vi "drawField.vi"(0 "Vision in":refnum<class "Vision.lvclass">, 1 "AutoScale":bool=TRUE, 2 "Game reference":refnum<data-value>, 5 "Field State Input":T1 {"Detection Frame Out"."robots_blue"."height" format="%+4.3f"; "Detection Frame Out"."robots_blue"."pixel_y" format="%+4.3f"; "Detection Frame Out"."robots_blue"."pixel_x" format="%+4.3f"; "Detection Frame Out"."robots_blue"."orientation" format="%+4.3f"; "Detection Frame Out"."robots_blue"."y" format="%+4.3f"; "Detection Frame Out"."robots_blue"."confidence" format="%4.3f"; "Detection Frame Out"."robots_blue"."x" format="%+4.3f"; "Detection Frame Out"."robots_yellow"."height" format="%+4.3f"; "Detection Frame Out"."robots_yellow"."pixel_y" format="%+4.3f"; "Detection Frame Out"."robots_yellow"."pixel_x" format="%+4.3f"; "Detection Frame Out"."robots_yellow"."orientation" format="%+4.3f"; "Detection Frame Out"."robots_yellow"."y" format="%+4.3f"; "Detection Frame Out"."robots_yellow"."confidence" format="%4.3f"; "Detection Frame Out"."robots_yellow"."x" format="%+4.3f"}, 11 "error in (no error)":errorcluster, 12 "Scale mm/pixel":dbl=0.094076928 format="%#_13g", 13 "Draw Targets?":T6, 14 "Zoom":dbl) -> (3 "AutoScale Out":bool=TRUE, 4 "Vision out":refnum<class "Vision.lvclass">, 6 "2D Picture":picture, 10 "Scale Out":dbl, 15 "error out":errorcluster)   [LabVIEW 2021, in "Vision.lvclass"]
uses:
  Vision.lvclass
  DrawTargets.ctl
  Controls/SSL Field State.ctl
  Controls/SSL Detection Frame.ctl
  Controls/SSL Detection Robot.ctl
  <vilib>/Analysis/Matrix/Datatypes/RealMatrix.ctl
  Controls/SSL Detection Ball.ctl
  Game_class/Game.lvclass
  <vilib>/Utility/miscctls.llb/LVBoundsTypeDef.ctl
  Robot_class/Robot.lvclass
  Game_class/Game.lvclass/Game.ctl
  Team_class/Team.lvclass/Team.ctl
  Parameters_class/Parameters.lvclass/Parameters.ctl
  Game_class/Read Referee.vi
  Game_class/Read OffensiveTeam.vi
  Game_class/Read DefensiveTeam.vi
  Game_class/Read KeeperTeam.vi
  Game_class/Read Parameters.lvclass.vi
  Game_class/Read FieldRef.vi
  Game_class/Read AllyRef.vi
  Game_class/Read EnemyRef.vi
  Game_class/Read BallRef.vi
  Team_class/Read RobotRef.vi
  Parameters_class/Read Area.vi
  Parameters_class/Read Project.vi
  Team_class/Read KeeperPlay.vi
  Ally_class/Ally.lvclass
  D:/RoboIme/horie/SSL_AI/Team_class/Team.lvclass
  Enemy_class/Enemy.lvclass
  Referee_class/Referee.lvclass
  Parameters_class/Parameters.lvclass
  Field_class/Field.lvclass
  Ball_class/Ball.lvclass
  <vilib>/Analysis/Matrix/NI_Matrix.lvlib
panel:
  in  "Defense stretch":i32=500
  in  "Draw Number":bool=TRUE
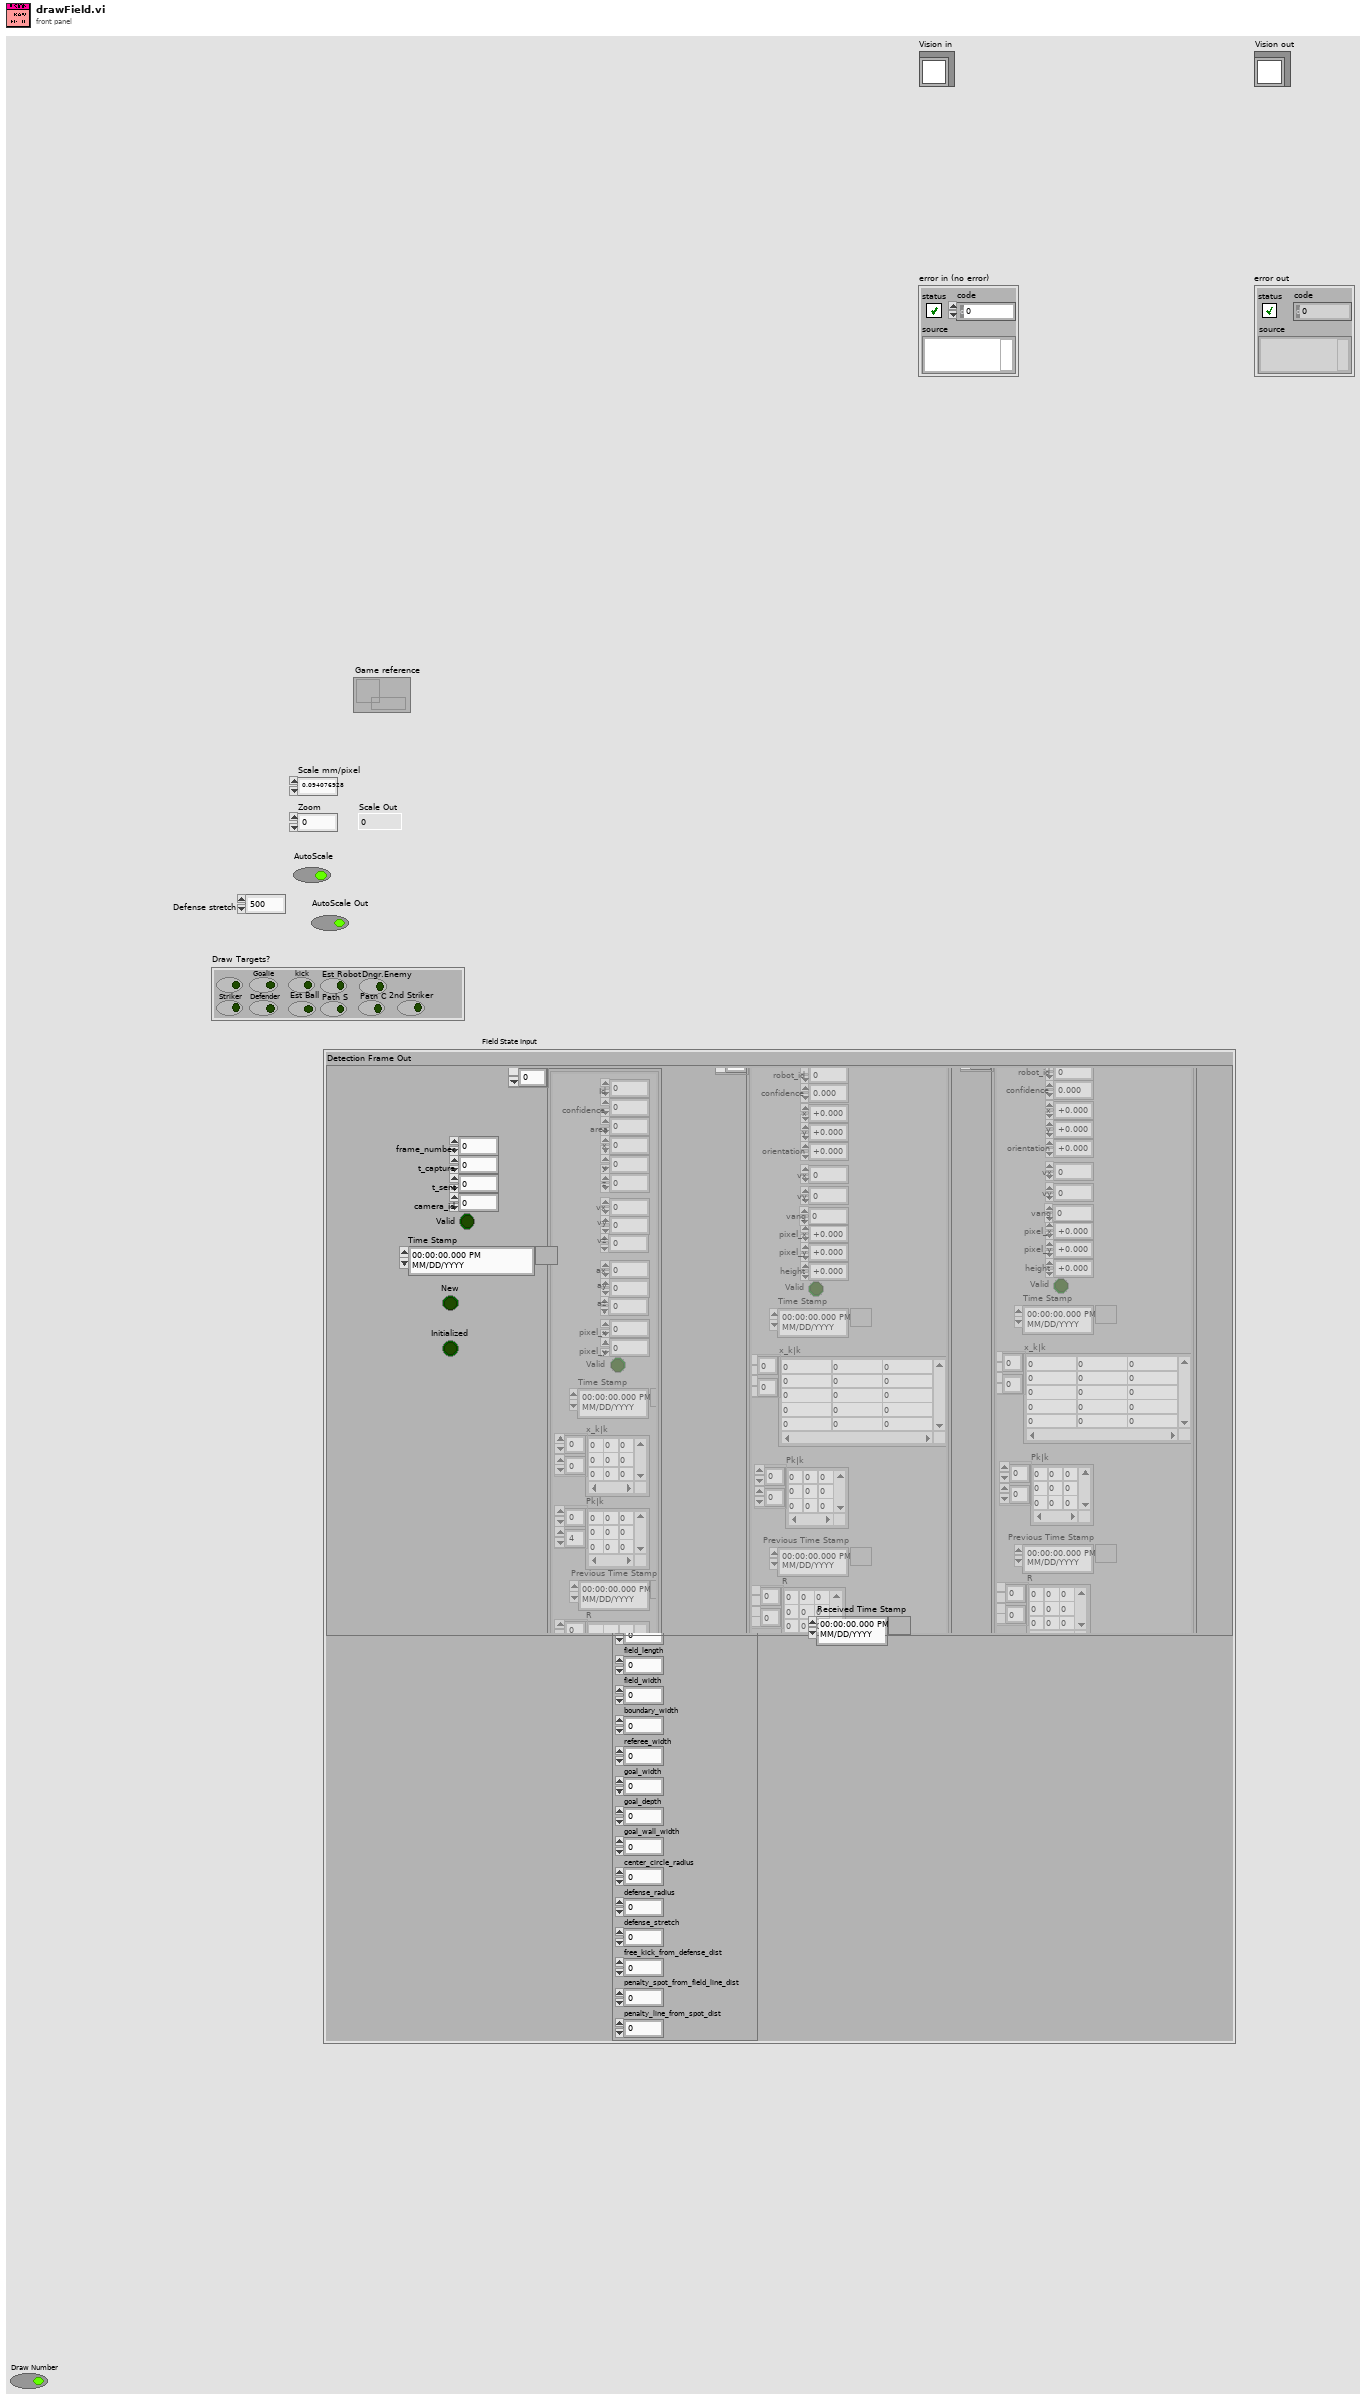
[diagram p1: front panel]
types:
  T1 = typedef "SSL Field State.ctl" = cluster{"Detection Frame Out":T2, "Field Size Out":cluster{"line_width":u32, "field_length":u32, "field_width":u32, "boundary_width":u32, "referee_width":u32, "goal_width":u32, "goal_depth":u32, "goal_wall_width":u32, "center_circle_radius":u32, "defense_radius":u32, "defense_stretch":u32, "free_kick_from_defense_dist":u32, "penalty_spot_from_field_line_dist":u32, "penalty_line_from_spot_dist":u32}, "Received Time Stamp":timestamp}
  T2 = typedef "SSL Detection Frame.ctl" = cluster{"frame_number":u32, "t_capture":dbl, "t_sent":dbl, "camera_id":u32, "robots_yellow":T3[], "robots_blue":T3[], "balls":T5[], "Valid":bool, "Time Stamp":timestamp, "New":bool, "Initialized":bool}
  T3 = typedef "SSL Detection Robot.ctl" = cluster{"x":sgl, "robot_id":u32, "confidence":sgl, "y":sgl, "orientation":sgl, "pixel_x":sgl, "pixel_y":sgl, "height":sgl, "Valid":bool, "Time Stamp":timestamp, "x_k|k":T4, "Pk|k":T4, "Previous Time Stamp":timestamp, "R":T4, "vx":dbl, "vy":dbl, "vang":dbl}
  T4 = typedef "NI_Matrix.lvlib/RealMatrix.ctl" = dbl[][]
  T5 = typedef "SSL Detection Ball.ctl" = cluster{"x":sgl, "area":u32, "confidence":sgl, "y":sgl, "z":sgl, "pixel_x":sgl, "pixel_y":sgl, "Valid":bool, "Time Stamp":timestamp, "x_k|k":T4, "Pk|k":T4, "Id":u32, "Previous Time Stamp":timestamp, "R":T4, " vx":sgl, "vy":dbl, "vz":dbl, " ax":sgl, "ay":dbl, "az":dbl}
  T6 = typedef "DrawTargets.ctl" = cluster{"Attacker":bool, "Striker":bool, "Goalie":bool, "Defender":bool, "kick":bool, "Est Ball":bool, "Est Robot":bool, "Path S":bool, "Path C":bool, "Dngr.Enemy":bool, "2nd Striker":bool}
  T7 = typedef "LVBoundsTypeDef.ctl" = cluster{"Width":u32, "Height":u32}
  T8 = typedef "Project.ctl" = enum16{"SSL", "VSS"}
  T9 = typedef "KeeperPlay.ctl" = enum16{"SimpleBallPlacementAlly", "BallPlacementAlly", "BallPlacementEnemy", "ZigZag", "Goto", "NormalGame", "KeeperPlay", "Halt", "Timeout", "PenaltyEnemy", "TestPlay"}
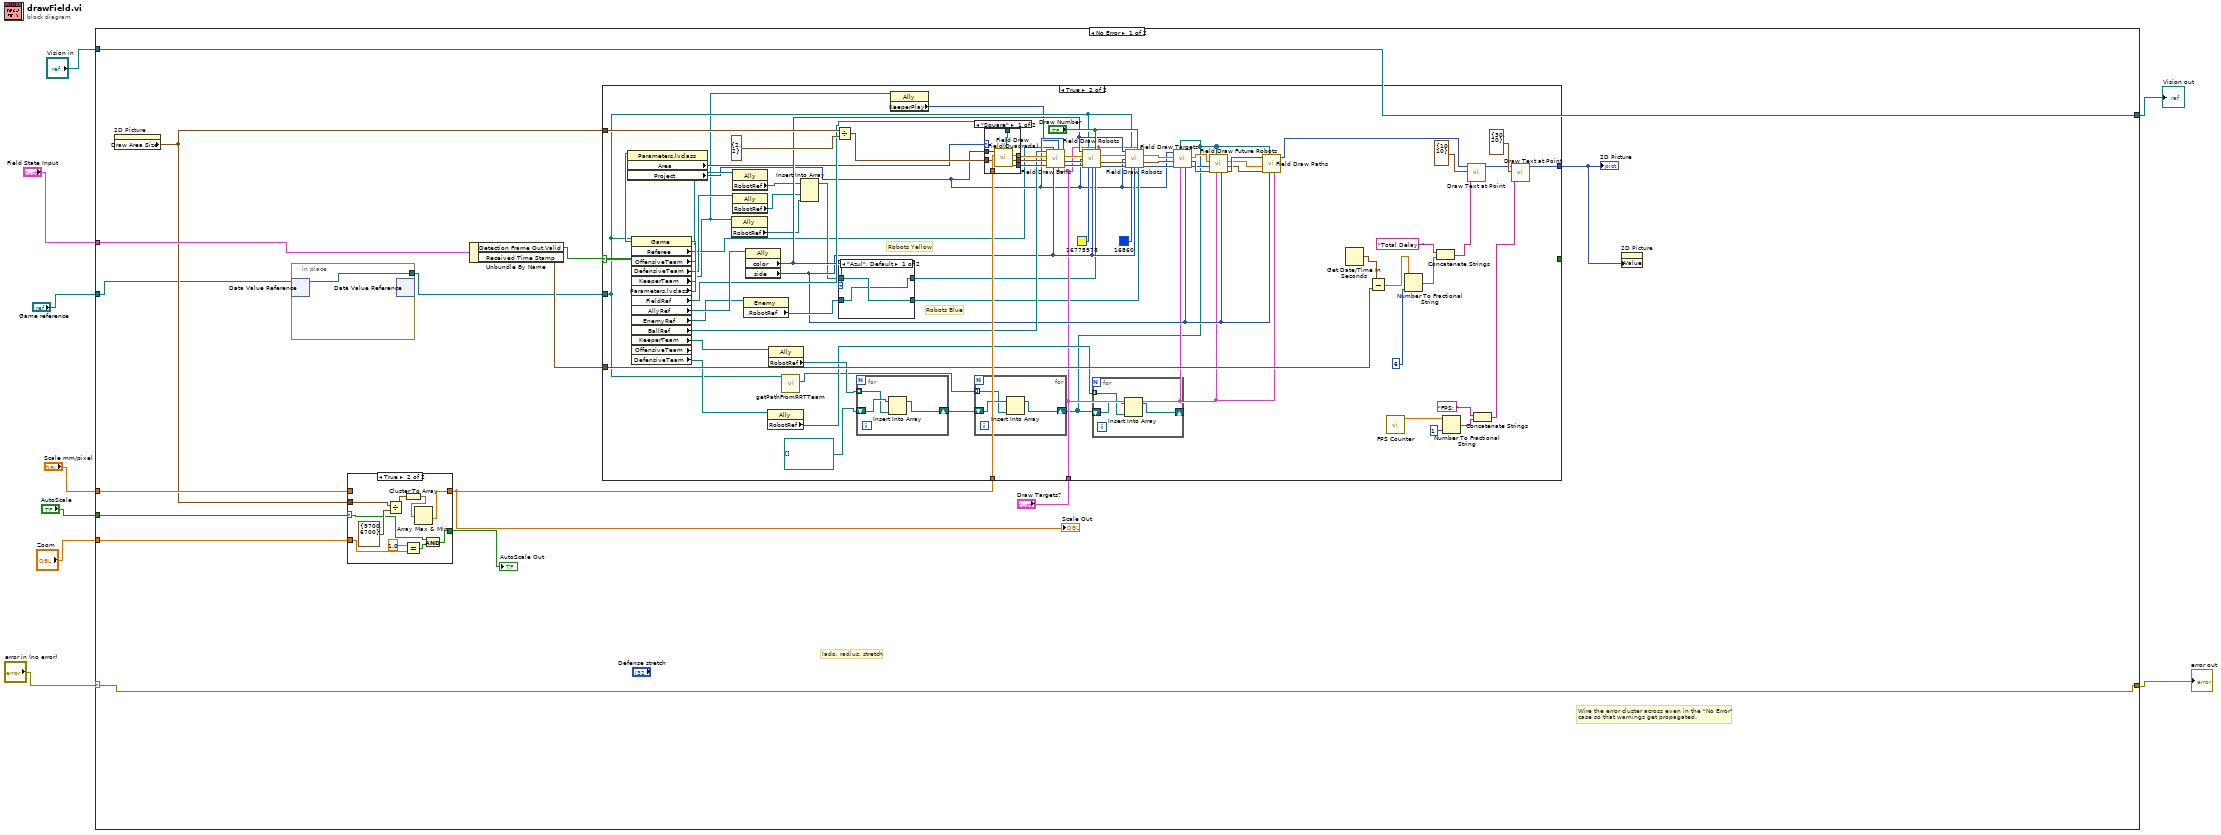
[diagram p0: block diagram]
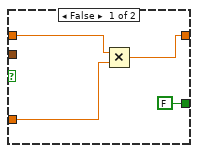
[diagram p2: hidden frame]
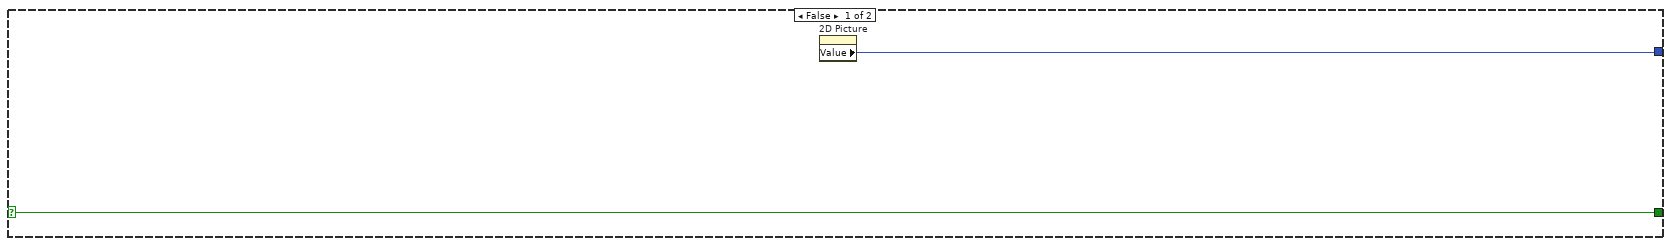
[diagram p3: hidden frame]
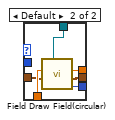
[diagram p5: hidden frame]
diagram:
  n1 = case shown="No Error" "error in (no error)" {
    selector: "error in (no error)" -> [w23 w142]
    tunnel: [w23 w142] -> w8
    tunnel: [w24 w141] -> w6
    tunnel: "Vision in" -> [w24 w141]
    tunnel: "Scale mm/pixel" -> [w20 _]
    tunnel: "AutoScale" -> [w19 _]
    tunnel: "Zoom" -> [w18 _]
    tunnel: "Field State Input" -> [w16 _]
    tunnel: "Game reference" -> [w13 _]
    frame No Error {
      # "lado, radius, stretch"
      # "Wire the error cluster across even in the \"No Error\"\ncase so that warnings get propagated."
      n2 = property on="2D Picture" class="Pict"() -> ("Draw Area Size"=w15:T7)  [unwired: 2 in, 2 out]
      n3 = in-place {
        in-place-border: [w25] -> w12
        n4 = in-place-dvr #1(w13) -> (w25:refnum<class "Game.lvclass">)  [unwired: 1 out]
        n5 = in-place-dvr #1() -> ()  [unwired: 1 in, 2 out]
      }
      n6 = case shown="True" w19 {
        selector: w19 -> [_ w31]
        tunnel: w20 -> [w29 _]
        tunnel: [w28 w35] -> w14
        tunnel: w15 -> [_ w39]
        tunnel: w18 -> [w27 w34]
        tunnel: [FALSE w32] -> w17
        frame False {
          n7 = Multiply(x=w29, y=w27) -> (x*y=w28:dbl)
        }
        frame True {
          n8 = Divide(x=w39, y=T7 {"Width"=9700, "Height"=6700}) -> (x/y=w37:cluster{"Width":dbl, "Height":dbl})
          n9 = Cluster To Array(cluster=w37) -> (array=w36:dbl[])
          n10 = Equal?(x=1.0, y=w34) -> (x = y?=w30:bool)
          n11 = Array Max & Min(array=w36) -> (min value=w35:dbl)  [unwired: 3 out]
          n12 = And(x=w31, y=w30) -> (x .and. y?=w32:bool)
        }
      }
      "Scale Out" <- w14
      "AutoScale Out" <- w17
      n13 = Unbundle By Name(w16) -> ("Detection Frame Out.Valid"=w11:bool, "Received Time Stamp"=w22:timestamp)
      n14 = case shown="True" w11 {
        selector: w11 -> [w41 _]
        tunnel: w15 -> [_ w113]
        tunnel: [w40 w94] -> w10
        tunnel: w14 -> [_ w106]
        tunnel: [w41 _] -> _
        tunnel: w22 -> [_ w101]
        tunnel: "Draw Targets?" -> [_ w59]
        tunnel: w12 -> [_ w46]
        frame False {
          n15 = property on="2D Picture" class="Pict"() -> ("Value"=w40:picture)  [unwired: 2 in, 2 out]
        }
        frame True {
          # "Robots Blue"
          # "Robots Yellow"
          n16 = property class="Game" props=["Referee", "OffensiveTeam", "DefensiveTeam", "KeeperTeam", "Parameters.lvclass", "FieldRef", "AllyRef", "EnemyRef", "BallRef", "KeeperTeam", "OffensiveTeam", "DefensiveTeam"](reference=w46) -> ("Referee"=w44:refnum<class "Referee.lvclass">, "OffensiveTeam"=w56:refnum<class "Ally.lvclass">, "DefensiveTeam"=w55:refnum<class "Ally.lvclass">, "KeeperTeam"=w43:refnum<class "Ally.lvclass">, "Parameters.lvclass"=w61:refnum<class "Parameters.lvclass">, "FieldRef"=w70:refnum<class "Field.lvclass">, "AllyRef"=w76:refnum<class "Ally.lvclass">, "EnemyRef"=w75:refnum<class "Enemy.lvclass">, "BallRef"=w73:refnum<class "Ball.lvclass">, "KeeperTeam"=w68:refnum<class "Ally.lvclass">, "DefensiveTeam"=w67:refnum<class "Ally.lvclass">)  [unwired: 1 in, 3 out]
          n17 = property class="Parameters.lvclass"(reference=w61) -> ("Area"=w60:enum16{"Circular", "Square"}, "Project"=w48:T8)  [unwired: 1 in, 2 out]
          n18 = property class="Ally"(reference=w43) -> ("RobotRef"=w52:refnum<class "Robot.lvclass">[])  [unwired: 1 in, 2 out]
          n19 = property class="Ally"(reference=w56) -> ("RobotRef"=w54:refnum<class "Robot.lvclass">[])  [unwired: 1 in, 2 out]
          n20 = property class="Ally"(reference=w55) -> ("RobotRef"=w53:refnum<class "Robot.lvclass">[])  [unwired: 1 in, 2 out]
          n21 = property class="Enemy"(reference=w75) -> ("RobotRef"=w74:refnum<class "Robot.lvclass">[])  [unwired: 1 in, 2 out]
          n22 = property class="Ally"(reference=w76) -> ("color"=w69:enum16{"Azul", "Amarelo"}, "side"=w62:enum16{"Esquerdo", "Direito"})  [unwired: 1 in, 2 out]
          n23 = property class="Ally"(reference=w67) -> ("RobotRef"=w63:refnum<class "Robot.lvclass">[])  [unwired: 1 in, 2 out]
          n24 = property class="Ally"(reference=w68) -> ("RobotRef"=w64:refnum<class "Robot.lvclass">[])  [unwired: 1 in, 2 out]
          n25 = call "getPathFromRRTTeam.vi"("Game in"=w46) -> ("RoboRef"=w47:refnum<class "Robot.lvclass">[])  [unwired: 8 in, 2 out]
          n26 = Insert Into Array(array=w54, new element #1=w53, new element #2=w52) -> (w51:refnum<class "Robot.lvclass">[])  [unwired: 1 in]
          n27 = Divide(x=w113, y=T7 {"Width"=2, "Height"=2}) -> (x/y=w104:cluster{"Width":dbl, "Height":dbl})
          n28 = case shown="\"Azul\", Default" w69 {
            tunnel: w74 -> [w124 w126]
            tunnel: [w124 w127] -> w50
            tunnel: w51 -> [w125 w127]
            tunnel: [w125 w126] -> w49
            frame "Azul", Default {
            }
            frame "Amarelo" {
            }
          }
          n29 = for {
            tunnel: w64 -> [w122] mode=indexing
            shift-right: [w121] -> w65
            shift-left: refnum<class "Robot.lvclass">[] [] ("RobotRef") -> [w123]
            n30 = Insert Into Array(array=w123, new element=w122) -> (w121:refnum<class "Robot.lvclass">[])  [unwired: 1 in]
          }
          n31 = property class="Ally"(reference=w43) -> ("KeeperPlay"=w42:T9)  [unwired: 1 in, 2 out]
          n32 = for {
            tunnel: w47 -> [w119] mode=indexing
            shift-right: [w118] -> w45
            shift-left: w65 -> [w120]
            n33 = Insert Into Array(array=w120, new element=w119) -> (w118:refnum<class "Robot.lvclass">[])  [unwired: 1 in]
          }
          n34 = case shown="\"Square\"" w60 {
            tunnel: w106 -> [w134 w140]
            tunnel: [w133 w139] -> w105
            tunnel: [w130 w136] -> w77
            tunnel: w104 -> [w132 w138]
            tunnel: [w131 w137] -> w103
            tunnel: w70 -> [w129 w135]
            tunnel: w48 -> [w128 _]
            frame "Square" {
              n35 = call "Field Draw Field(Quadrada).vi"("FieldRef"=w129, "Offset"=w132, "Scale"=w134, "Project"=w128) -> ("new picture out"=w130:picture, "Offset Out"=w131:cluster{"Width":dbl, "Height":dbl}, "Scale Out"=w133:dbl)  [unwired: 5 in]
            }
            frame Default {
              n36 = call "Field Draw Field(circular).vi"("FieldRef"=w135, "Offset"=w138, "Scale"=w140) -> ("new picture out"=w136:picture, "Offset Out"=w137:cluster{"Width":dbl, "Height":dbl}, "Scale Out"=w139:dbl)  [unwired: 6 in]
            }
          }
          n37 = call "Field Draw Balls.vi"("Project"=w48, "Draw Targets?"=w59, "KeeperPlay"=w42, "side"=w62, "Referee"=w44, "Picture In"=w77, "Offset"=w103, "Scale"=w105, "BallRef"=w73) -> ("Picture Out"=w112:picture, "Offset Out"=w72:cluster{"Width":dbl, "Height":dbl}, "Scale Out"=w111:dbl)
          n38 = call "Field Draw Robots.vi"("color"=w69, "game in"=w46, "Draw Number"="Draw Number", "Draw Targets?"=w59, "Scale"=w111, "Project"=w48, "Offset"=w72, "Picture In"=w112, "color(black)"=u32 16775978, "Lado"=w62, "RobotRef"=w50) -> ("Scale Out"=w110:dbl, "Offset Out"=w109:cluster{"Width":dbl, "Height":dbl}, "Picture Out"=w108:picture)  [unwired: 2 in]
          n39 = for {
            tunnel: w63 -> [w116] mode=indexing
            shift-right: [w115] -> _
            shift-left: w45 -> [w117]
            n40 = Insert Into Array(array=w117, new element=w116) -> (w115:refnum<class "Robot.lvclass">[])  [unwired: 1 in]
          }
          n41 = call "Field Draw Robots.vi"("color"=w69, "game in"=w46, "Draw Number"="Draw Number", "Draw Targets?"=w59, "Scale"=w110, "Project"=w48, "Offset"=w109, "Picture In"=w108, "color(black)"=u32 16860, "Lado"=w62, "RobotRef"=w49) -> ("Scale Out"=w85:dbl, "Offset Out"=w86:cluster{"Width":dbl, "Height":dbl}, "Picture Out"=w58:picture)  [unwired: 2 in]
          n42 = call "Field Draw Targets.vi"("Lado"=w62, "Draw Targets?"=w59, "RobotRef"=w45, "Picture In"=w58, "Offset"=w86, "Scale"=w85, "Project"=w48) -> ("Picture Out"=w57:picture, "Offset Out"=w84:cluster{"Width":dbl, "Height":dbl}, "Scale Out"=w83:dbl)  [unwired: 2 in]
          n43 = call "Field Draw Future Robots.vi"("Lado"=w62, "Draw Targets?"=w59, "RobotRef"=w45, "Offset"=w84, "Picture In"=w57, "Scale"=w83) -> ("Picture Out"=w81:picture, "Offset Out"=w79:cluster{"Width":dbl, "Height":dbl}, "Scale Out"=w80:dbl)  [unwired: 3 in]
          n44 = call "Field Draw Paths.vi"("Draw Targets?"=w59, "Lado"=w62, "RobotRef"=w45, "Offset"=w79, "Scale mm/pixel"=w80, "picture in"=w81) -> ("picture out"=w78:picture)  [unwired: 5 in]
          n45 = Get Date/Time In Seconds() -> (seconds since 1Jan1904=w100:timestamp)
          n46 = Subtract(x=w100, y=w101) -> (x-y=w99:dbl)
          n47 = call "FPS Counter.vi"() -> ("FPS"=w90:dbl)  [unwired: 11 in]
          n48 = Number To Fractional String(number=w99, precision (6)=i16 6) -> (F-format string=w97:string)  [unwired: 2 in]
          n49 = Concatenate Strings("Total Delay: " ("text"), w97) -> (w96:string)
          n50 = Number To Fractional String(number=w90, precision (6)=i16 1) -> (F-format string=w92:string)  [unwired: 2 in]
          n51 = call <vilib>:"Draw Text at Point.vi"("text"=w96, "origin"=cluster{"x":i16, "y":i16} {"x"=10, "y"=10}, "picture"=w78) -> ("new picture"=w82:picture)  [unwired: 7 in, 1 out]
          n52 = Concatenate Strings("FPS: " ("text"), w92) -> (w88:string)
          n53 = call <vilib>:"Draw Text at Point.vi"("text"=w88, "origin"=cluster{"x":i16, "y":i16} {"x"=30, "y"=20}, "picture"=w82) -> ("new picture"=w94:picture)  [unwired: 7 in, 1 out]
        }
      }
      "2D Picture" <- w10
      n54 = property on="2D Picture" class="Pict"("Value"=w10) -> ()  [unwired: 2 in, 2 out]
    }
    frame Error {
    }
  }
  "error out" <- w8
  "Vision out" <- w6
